vi "Show Windows System(Lot Start).vi"(0 "vi reference in":refnum<vi>, 5 "Show":bool=TRUE, 7 "目前工站號":u8=1, 11 "_error In":errorcluster) -> (4 "vi reference out":refnum<vi>, 6 "Selection Result":enum16{"Nothing", "OK", "Cancel"}(ring), 8 "是否已入Tray 2":bool, 10 "生產數量 2":i32 max=5, 13 "目前工站號 2":u8=1, 14 "工站 2":T1={"工站1"=TRUE, "工站2"=TRUE, "工站3"=TRUE, "工站4"=TRUE, "工站5"=TRUE, "工站6"=TRUE, "工站7"=TRUE, "工站8"=TRUE}, 15 "_error out":errorcluster)   [LabVIEW 2015]
panel:
  in  "工站":T1={"工站1"=TRUE, "工站2"=TRUE, "工站3"=TRUE, "工站4"=TRUE, "工站5"=TRUE, "工站6"=TRUE, "工站7"=TRUE, "工站8"=TRUE}
  in  "是否已入Tray":bool
  in  "生產數量":i32 max=9999
  in  "Cancel Button":bool
  in  "OK Button":bool
  in  "Check":bool=TRUE
  # "開始生產,請輸入數量\n(若輸入 \"0\" , 則不限生產數量)"
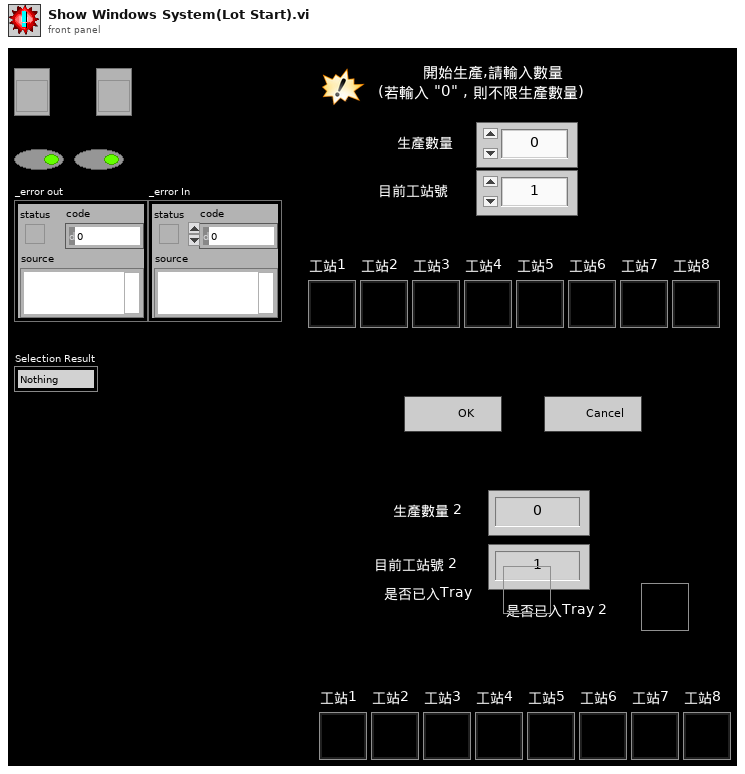
[diagram p1: front panel]
types:
  T1 = cluster{"工站1":bool, "工站2":bool, "工站3":bool, "工站4":bool, "工站5":bool, "工站6":bool, "工站7":bool, "工站8":bool}
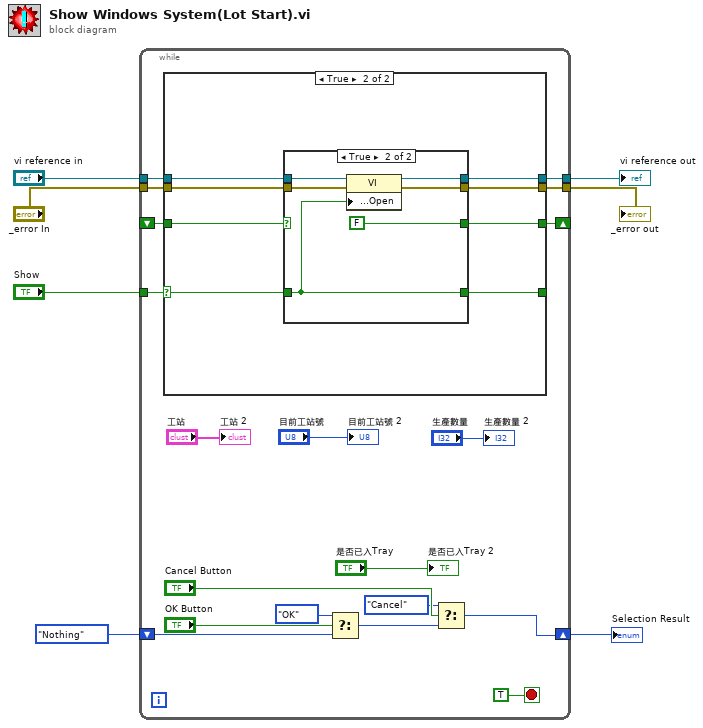
[diagram p0: block diagram]
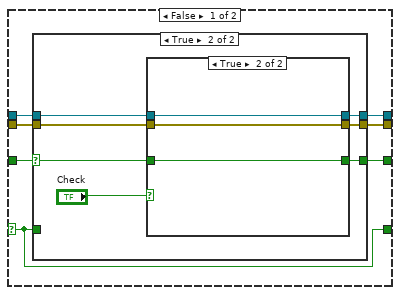
[diagram p2: hidden frame]
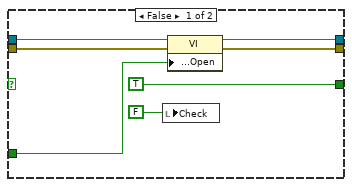
[diagram p3: hidden frame]
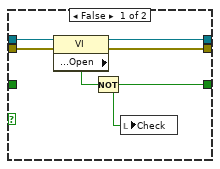
[diagram p4: hidden frame]
diagram:
  n1 = while {
    shift-right: [w22] -> _
    shift-left: _ -> [w21]
    tunnel: "Show" -> [w12]
    tunnel: "vi reference in" -> [w26]
    tunnel: "_error In" -> [w25]
    tunnel: [w24] -> w4
    tunnel: [w23] -> w3
    shift-right: [w15] -> w1
    shift-left: enum16{"Nothing", "OK", "Cancel"}."Nothing" ("Selection Result") -> [w14]
    stop <- TRUE ("Boolean 2") stop-if-true
    n2 = case shown="True" w12 {
      selector: w12 -> [w27 w58]
      tunnel: w26 -> [w33 w64]
      tunnel: w25 -> [w32 w63]
      tunnel: [w31 w62] -> w24
      tunnel: [w30 w61] -> w23
      tunnel: [w28 w60] -> w22
      tunnel: w21 -> [w29 w59]
      tunnel: [w27 w57] -> _
      frame False {
        n3 = case shown="True" w29 {
          selector: w29 -> [_ w41]
          tunnel: w33 -> [w40 w47]
          tunnel: w32 -> [w39 w46]
          tunnel: [w38 w45] -> w31
          tunnel: [w37 w44] -> w30
          tunnel: [TRUE w42] -> w28
          tunnel: w27 -> [w35 _]
          frame False {
            n4 = local write "Check"(FALSE ("Check")) -> ()
            n5 = property class="VI"(reference=w40, error in=w39, "Front Panel.Open"=w35) -> (reference out=w38:refnum<vi>, error out=w37:errorcluster)
          }
          frame True {
            n6 = case shown="True" "Check" {
              tunnel: w47 -> [w53 w55]
              tunnel: w46 -> [w52 w54]
              tunnel: [w51 w55] -> w45
              tunnel: [w50 w54] -> w44
              tunnel: [w48 w56] -> w42
              tunnel: w41 -> [_ w56]
              frame False {
                n7 = property class="VI"(reference=w53, error in=w52) -> (reference out=w51:refnum<vi>, error out=w50:errorcluster, "Front Panel.Open"=w49:bool)
                n8 = Not(x=w49) -> (.not. x?=w48:bool)
                n9 = local write "Check"(w48) -> ()
              }
              frame True {
              }
            }
          }
        }
      }
      frame True {
        n10 = case shown="True" w59 {
          selector: w59 -> [w68 _]
          tunnel: w64 -> [w67 w74]
          tunnel: w63 -> [w66 w73]
          tunnel: [w67 w72] -> w62
          tunnel: [w66 w71] -> w61
          tunnel: [w68 FALSE] -> w60
          tunnel: w58 -> [w65 w69]
          tunnel: [w65 w69] -> w57
          frame False {
          }
          frame True {
            n11 = property class="VI"(reference=w74, error in=w73, "Front Panel.Open"=w69) -> (reference out=w72:refnum<vi>, error out=w71:errorcluster)
          }
        }
      }
    }
    n12 = Select(t=enum16{"Nothing", "OK", "Cancel"}."OK" ("Selection Result"), s="OK Button", f=w14) -> (s? t:f=w19:enum16{"Nothing", "OK", "Cancel"})
    n13 = Select(t=enum16{"Nothing", "OK", "Cancel"}."Cancel" ("Selection Result"), s="Cancel Button", f=w19) -> (s? t:f=w15:enum16{"Nothing", "OK", "Cancel"})
    "生產數量 2" <- "生產數量"
    "目前工站號 2" <- "目前工站號"
    "是否已入Tray 2" <- "是否已入Tray"
    "工站 2" <- "工站"
  }
  "_error out" <- w3
  "vi reference out" <- w4
  "Selection Result" <- w1
